vi "FTW-ERR-ThrowInfo.vi"(7 "Informational Message":string, 11 "error in":errorcluster) -> (15 "error out":errorcluster)   [LabVIEW 2014]
panel:
  # "Inputs"
  # "Outputs"
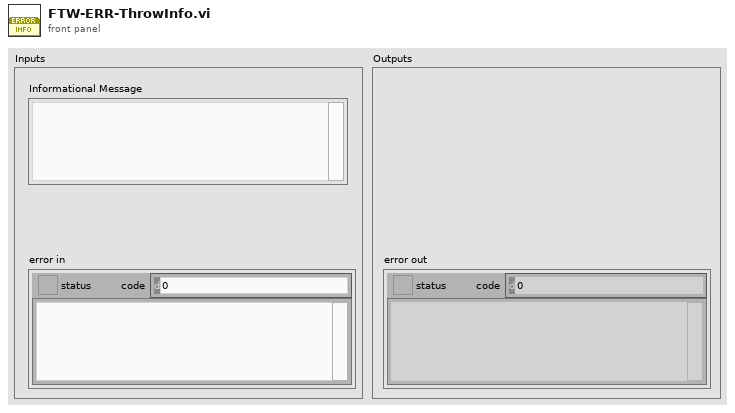
[diagram p1: front panel]
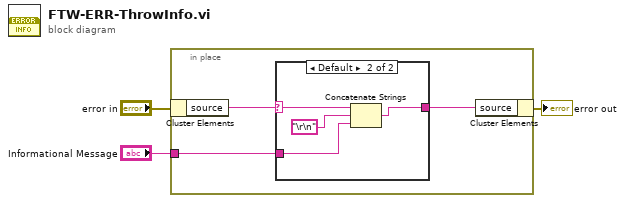
[diagram p0: block diagram]
diagram:
  n1 = in-place {
    in-place-border: "Informational Message" -> [w5]
    n2 = in-place-cluster #1("error in") -> ("source"=w4:string)
    n3 = case shown="Default" w4 {
      selector: w4 -> [_ w8]
      tunnel: [w7 w11] -> w6
      tunnel: w5 -> [w7 w9]
      frame "\u0000" {
      }
      frame Default {
        n4 = Concatenate Strings(w8, "\r\n", w9) -> (w11:string)
      }
    }
    n5 = in-place-cluster #1("source"=w6) -> (→"error out":errorcluster)
  }
